vi "Calculate Expected Panel Output.vi"(11 "PanelTestData":cluster{"Temperature":dbl, "LightIntensity":dbl}) -> (3 "Expected Result":dbl)   [LabVIEW 2013]
doc: "Calculates the voltage that the solar panel should produce at given conditions using a mathmatical algorithm."
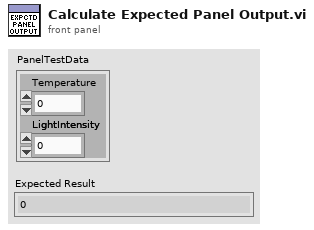
[diagram p1: front panel]
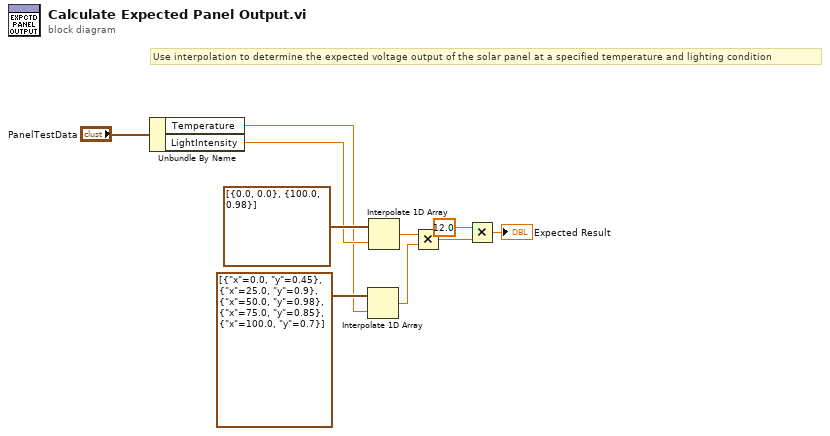
[diagram p0: block diagram]
diagram:
  # "Use interpolation to determine the expected voltage output of the solar panel at a specified temperature and lighting condition"
  n1 = Unbundle By Name("PanelTestData") -> ("Temperature"=w3:dbl, "LightIntensity"=w5:dbl)
  n2 = Interpolate 1D Array(1:w3, 2:cluster{"x":dbl, "y":dbl}[] [{"x"=0.0, "y"=0.45}, {"x"=25.0, "y"=0.9}, {"x"=50.0, "y"=0.98}, {"x"=75.0, "y"=0.85}, {"x"=100.0, "y"=0.7}] ("array of numbers or points")) -> (0:w2:dbl)
  n3 = Interpolate 1D Array(1:w5, 2:cluster{dbl, dbl}[] [{0.0, 0.0}, {100.0, 0.98}] ("array of numbers or points")) -> (0:w1:dbl)
  n4 = Multiply(x=w1, y=w2) -> (x*y=w9:dbl)
  n5 = Multiply(x=12.0, y=w9) -> (x*y=→"Expected Result":dbl)
